vi "Close Transport.vi"(8 "error in (no error)":errorcluster, 11 "ITransport in":refnum<class "ITransport.lvclass">) -> (0 "error out":errorcluster)   [LabVIEW 2017, in "ITransport.lvclass"]
uses:
  ITransport.lvclass
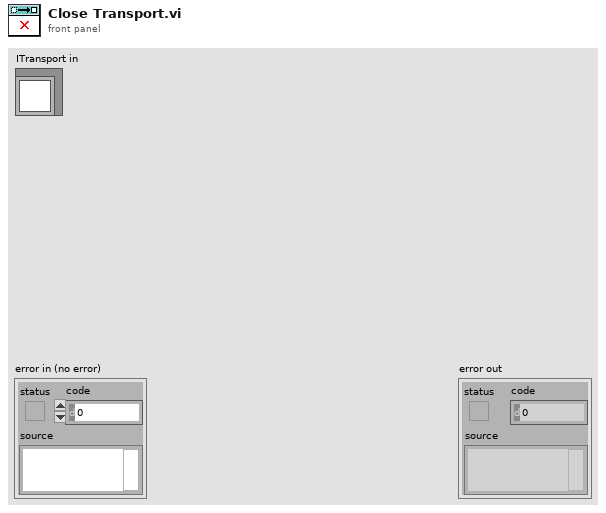
[diagram p1: front panel]
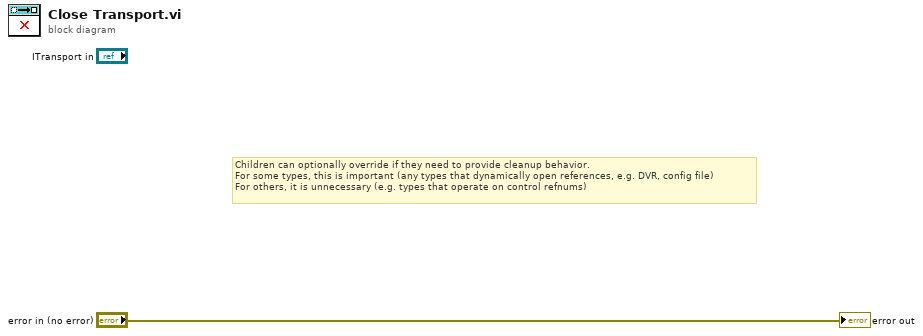
[diagram p0: block diagram]
diagram:
  # "Children can optionally override if they need to provide cleanup behavior.\nFor some types, this is important (any types that dynamically open references, e.g. DVR, config file)\nFor others, it is unnecessary (e.g. types that operate on control refnums)"
  "error out" <- "error in (no error)"
